vi "Queue Message Handler.vi"   [LabVIEW 2020]
uses:
  SubVI/Queue Create.vi
  SubVI/Queue Valid.vi
  SubVI/Queue Lossy Insert.vi
  SubVI/Queue Remove.vi
  SubVI/Queue Destroy.vi
panel:
  # "生产者\n消费者\n结构"
types:
  T1 = cluster{"Error":errorcluster, "Exit":bool, "queue":string, "data":variant}
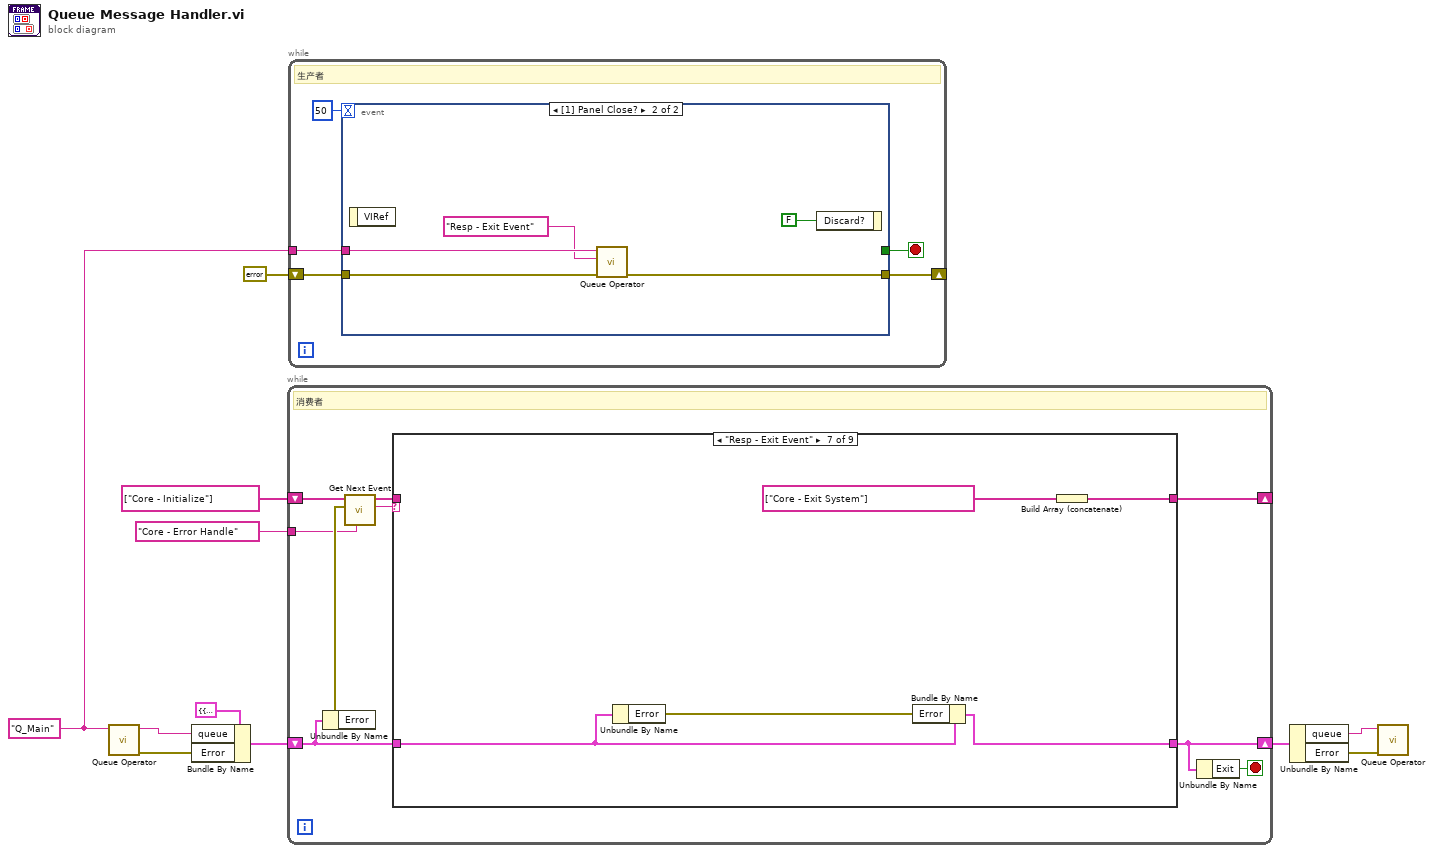
[diagram p0: block diagram]
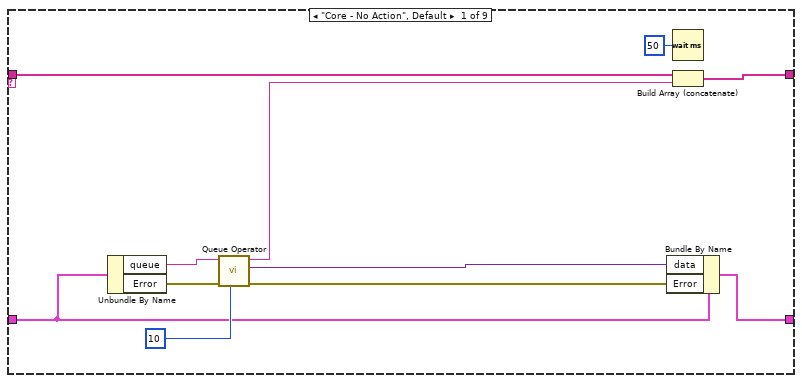
[diagram p2: hidden frame]
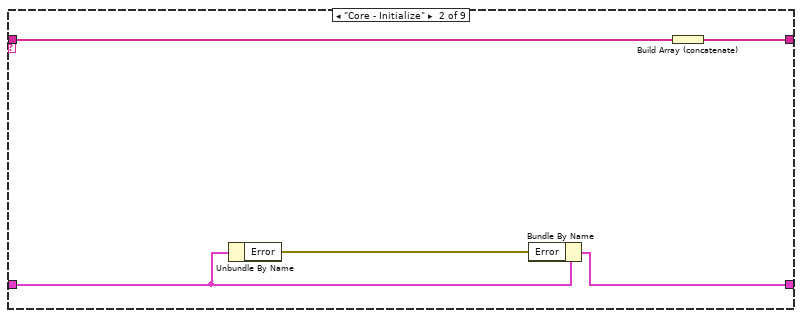
[diagram p3: hidden frame]
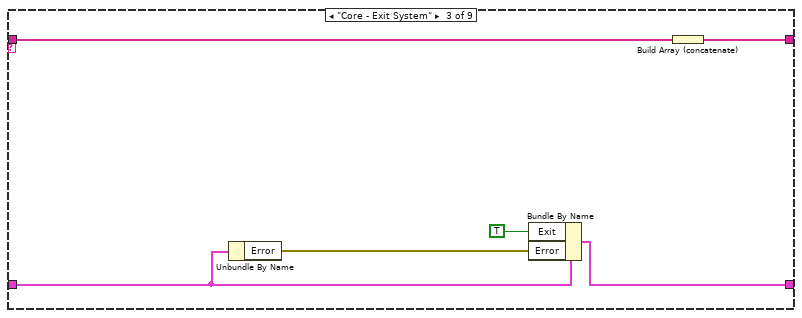
[diagram p4: hidden frame]
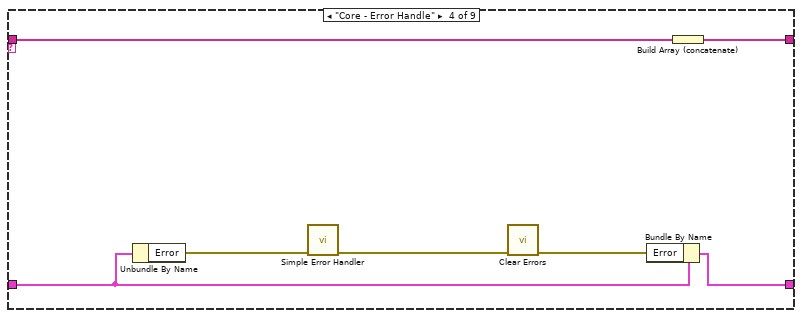
[diagram p5: hidden frame]
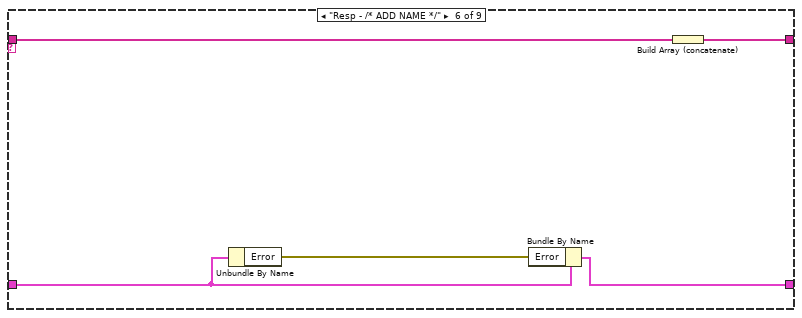
[diagram p7: hidden frame]
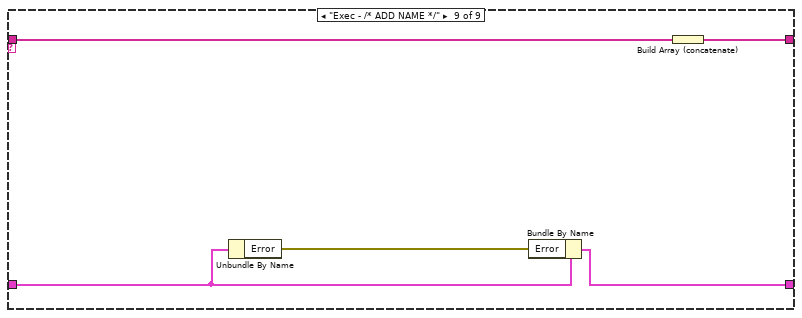
[diagram p9: hidden frame]
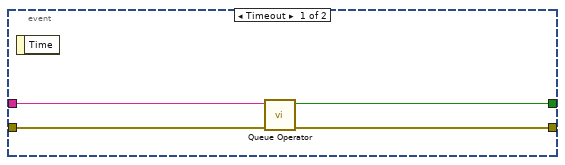
[diagram p10: hidden frame]
diagram:
  w3 = "Q_Main" ("queue name in")
  n1 = call-poly "Queue Operator.vi"("queue name in"=w3) -> ("error out"=w5:errorcluster, "queue name out"=w4:string)  [unwired: 7 in, 2 out]
  n2 = Bundle By Name(cluster=T1 {"Error"={"status"=FALSE, "code"=0, "source"=""}, "Exit"=FALSE, "queue"="", "data"=variant} ("Temp Variable"), "queue"=w4, "Error"=w5) -> (w9:T1)
  n3 = while {
    shift-right: [w15] -> _
    shift-left: string[] ["Core - Initialize"] -> [w18]
    shift-right: [w14] -> w8
    shift-left: w9 -> [w17]
    tunnel: "Core - Error Handle" ("Error Handle") -> [w12]
    stop <- w13 stop-if-true
    # "消费者"
    n4 = Unbundle By Name(w17) -> ("Error"=w16:errorcluster)
    n5 = call "Get Next Event.vi"("Error Handle"=w12, "error in (no error)"=w16, "event queue in"=w18) -> ("next event"=w19:string, "event queue out"=w20:string[])  [unwired: 7 in]
    n6 = case shown="\"Resp - Exit Event\"" w19 {
      tunnel: w20 -> [w28 w36 w42 w49 w51 w56 _ w63 w68]
      tunnel: w17 -> [w26 w34 w40 w47 w50 w54 w60 w62 w66]
      tunnel: [w27 w35 w41 w48 w51 w55 w61 w63 w67] -> w15
      tunnel: [w24 w32 w39 w46 w50 w53 w59 w62 w65] -> w14
      frame "Core - No Action", Default {
        n7 = Unbundle By Name(w26) -> ("queue"=w30:string, "Error"=w31:errorcluster)
        n8 = call-poly "Queue Operator.vi"("timeout(ms: -1)"=10, "error in (no error)"=w31, "queue name"=w30) -> ("error out"=w25:errorcluster, "data"=w22:variant, "event"=w23:string)  [unwired: 5 in, 1 out]
        n9 = Bundle By Name(cluster=w26, "data"=w22, "Error"=w25) -> (w24:T1)
        n10 = Wait (ms)(milliseconds to wait=u32 50 ("等待时间（毫秒）")) -> ()  [unwired: 1 out]
        n11 = Build Array (concatenate)(w28, w23) -> (w27:string[])
      }
      frame "Core - Initialize" {
        n12 = Unbundle By Name(w34) -> ("Error"=w33:errorcluster)
        n13 = Bundle By Name(cluster=w34, "Error"=w33) -> (w32:T1)
        n14 = Build Array (concatenate)(w36) -> (w35:string[])
      }
      frame "Core - Exit System" {
        n15 = Unbundle By Name(w40) -> ("Error"=w38:errorcluster)
        n16 = Bundle By Name(cluster=w40, "Exit"=TRUE, "Error"=w38) -> (w39:T1)
        n17 = Build Array (concatenate)(w42) -> (w41:string[])
      }
      frame "Core - Error Handle" {
        n18 = Unbundle By Name(w47) -> ("Error"=w45:errorcluster)
        n19 = call <vilib>:"Simple Error Handler.vi"("error in (no error)"=w45) -> ("error out"=w43:errorcluster)  [unwired: 4 in, 4 out]
        n20 = call <vilib>:"Clear Errors.vi"("error in (no error)"=w43) -> ("error out"=w44:errorcluster)  [unwired: 5 in, 1 out]
        n21 = Bundle By Name(cluster=w47, "Error"=w44) -> (w46:T1)
        n22 = Build Array (concatenate)(w49) -> (w48:string[])
      }
      frame "---------------------------------Response---------------------------------" {
      }
      frame "Resp - /* ADD NAME */" {
        n23 = Unbundle By Name(w54) -> ("Error"=w52:errorcluster)
        n24 = Bundle By Name(cluster=w54, "Error"=w52) -> (w53:T1)
        n25 = Build Array (concatenate)(w56) -> (w55:string[])
      }
      frame "Resp - Exit Event" {
        n26 = Unbundle By Name(w60) -> ("Error"=w58:errorcluster)
        n27 = Bundle By Name(cluster=w60, "Error"=w58) -> (w59:T1)
        n28 = Build Array (concatenate)(string[] ["Core - Exit System"]) -> (w61:string[])
      }
      frame "----------------------------------Execute-----------------------------------" {
      }
      frame "Exec - /* ADD NAME */" {
        n29 = Unbundle By Name(w66) -> ("Error"=w64:errorcluster)
        n30 = Bundle By Name(cluster=w66, "Error"=w64) -> (w65:T1)
        n31 = Build Array (concatenate)(w68) -> (w67:string[])
      }
    }
    n32 = Unbundle By Name(w14) -> ("Exit"=w13:bool)
  }
  n33 = while {
    tunnel: w3 -> [w72]
    shift-right: [w70] -> _
    shift-left: errorcluster {"status"=FALSE, "code"=0, "source"=""} ("error constant") -> [w71]
    stop <- w69 stop-if-true
    # "生产者"
    n34 = event shown="[1] Panel Close?" {
      selector: _ -> [_ _]
      dyn-events: _ -> [_ _]
      timeout: 50 -> [_ _]
      tunnel: w72 -> [w76 w80]
      tunnel: w71 -> [w77 w81]
      tunnel: [w75 w79] -> w70
      tunnel: [w74 _] -> w69
      event Timeout {
        n35 = event-data() -> ()  [unwired: 1 in, 1 out]
        n36 = call-poly "Queue Operator.vi"("error in (no error)"=w77, "queue name in"=w76) -> ("error out"=w75:errorcluster, "invalid？"=w74:bool)  [unwired: 8 in]
      }
      event Panel Close? {
        n37 = event-data() -> ()  [unwired: 1 in, 1 out]
        n38 = call-poly "Queue Operator.vi"("error in (no error)"=w81, "event"="Resp - Exit Event", "queue name"=w80) -> ("error out"=w79:errorcluster)  [unwired: 6 in, 2 out]
        n39 = event-data("Discard?"=FALSE) -> ()  [unwired: 1 in, 1 out]
      }
    }
  }
  n40 = Unbundle By Name(w8) -> ("queue"=w6:string, "Error"=w7:errorcluster)
  n41 = call-poly "Queue Operator.vi"("error in (no error)"=w7, "queue name in"=w6) -> ()  [unwired: 8 in, 2 out]
